vi "Copy file to network and group server.vi"(10 "Overwrite existing file?":bool, 11 "File path in":path) -> (2 "Server error?":bool)   [LabVIEW 2011]
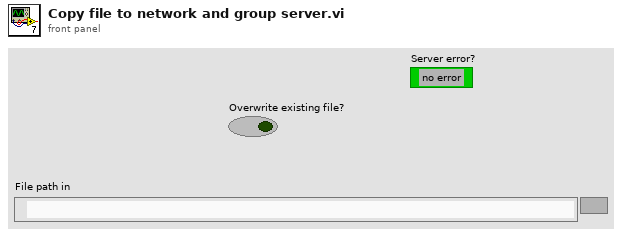
[diagram p1: front panel]
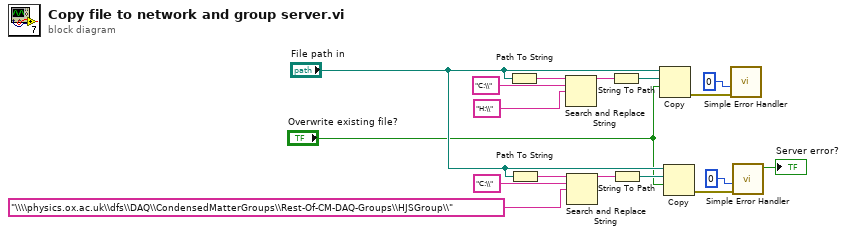
[diagram p0: block diagram]
diagram:
  n1 = Path To String(path="File path in") -> (string=w16:string)
  n2 = Path To String(path="File path in") -> (string=w11:string)
  n3 = Search and Replace String(input string=w16, search string="C:\\", replace string="H:\\") -> (result string=w17:string)  [unwired: 5 in, 3 out]
  n4 = Search and Replace String(input string=w11, search string="C:\\", replace string="\\\\physics.ox.ac.uk\\dfs\\DAQ\\CondensedMatterGroups\\Rest-Of-CM-DAQ-Groups\\HJSGroup\\") -> (result string=w13:string)  [unwired: 5 in, 3 out]
  n5 = String To Path(string=w17) -> (path=w5:path)
  n6 = String To Path(string=w13) -> (path=w12:path)
  n7 = Copy(9:"Overwrite existing file?", 10:w5, 11:"File path in") -> (0:w7:errorcluster)  [unwired: 2 in, 2 out]
  n8 = Copy(9:"Overwrite existing file?", 10:w12, 11:"File path in") -> (0:w3:errorcluster)  [unwired: 2 in, 2 out]
  n9 = call <vilib>:"Simple Error Handler.vi"("type of dialog (OK msg:1)"=0, "error in (no error)"=w7) -> ()  [unwired: 3 in, 5 out]
  n10 = call <vilib>:"Simple Error Handler.vi"("type of dialog (OK msg:1)"=0, "error in (no error)"=w3) -> ("error?"=→"Server error?":bool)  [unwired: 3 in, 4 out]
